vi "RPC Method package_service_method.vi"(8 "error in (no error)":errorcluster, 11 "ServiceName Template in":refnum<class "ServiceName Template.lvclass">) -> (0 "error out":errorcluster, 3 "ServiceName Template out":refnum<class "ServiceName Template.lvclass">)   [LabVIEW 2024, in "ServiceName Template.lvclass"]
uses:
  ServiceName Template.lvclass
  C:/serenial/oss/grpc-labview/labview source/gRPC lv Servicer/ServiceBase/ServiceBase.lvclass
  ServiceName Template.lvclass/ServiceName Template.ctl
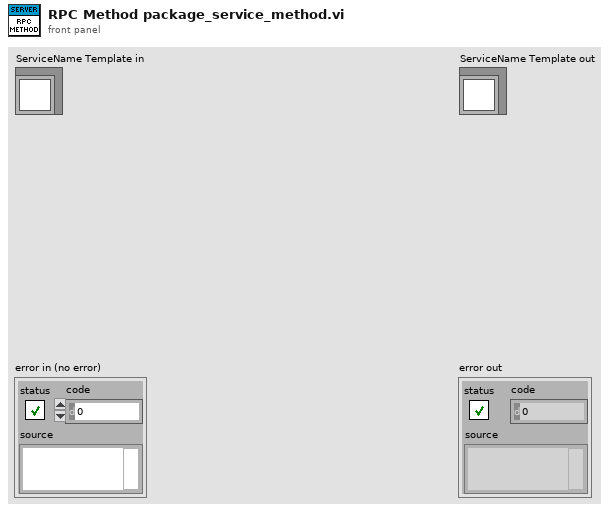
[diagram p1: front panel]
types:
  T1 = typedef "ServiceName Template.lvclass/Server Internal UEs.ctl" = cluster{"package_service_method Internal UE":refnum<user-event>}
  T2 = typedef "ServiceName Template.lvclass/Server gRPC UEs.ctl" = cluster{"package_service_method":refnum<user-event>}
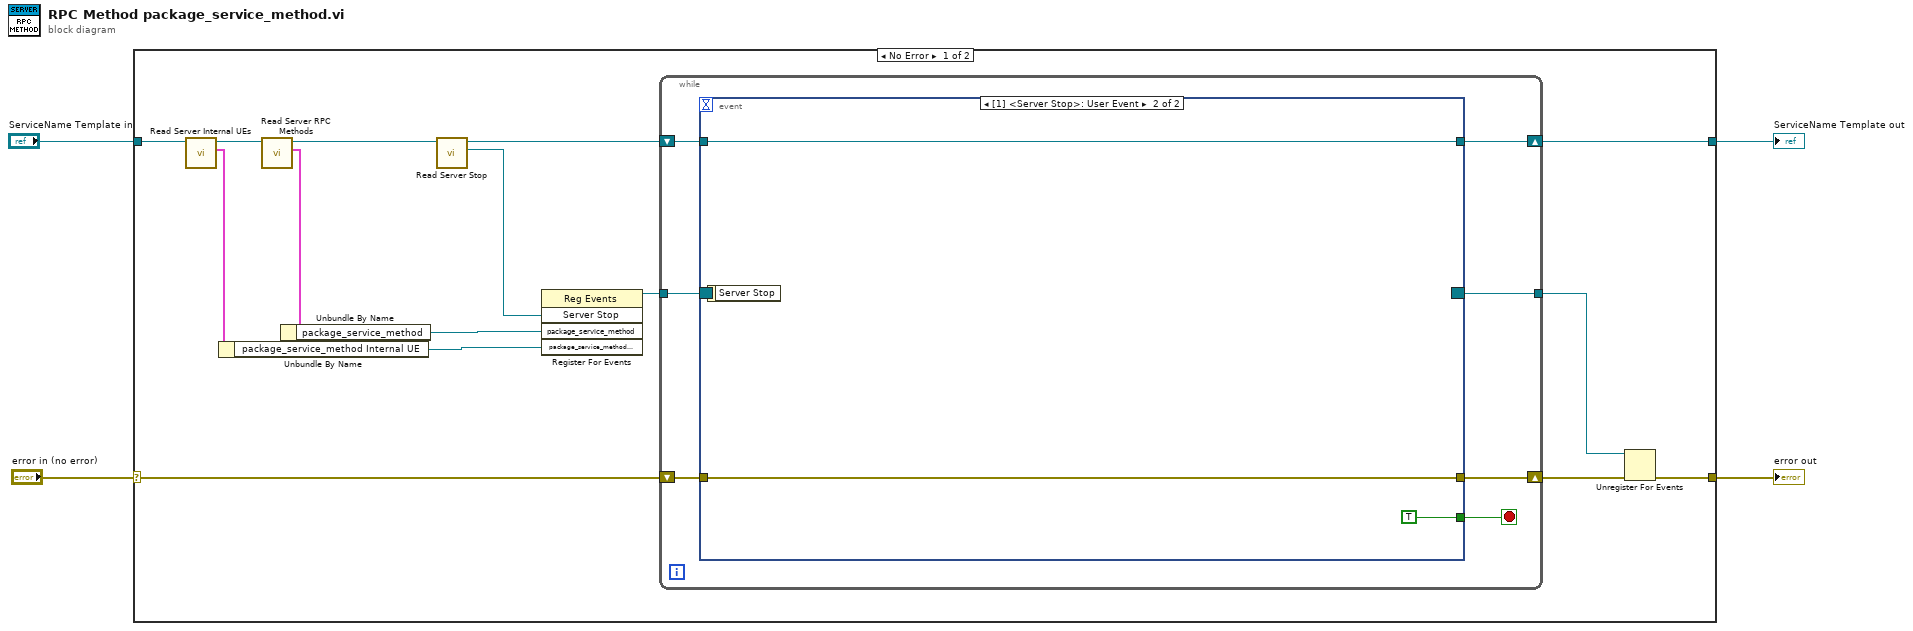
[diagram p0: block diagram]
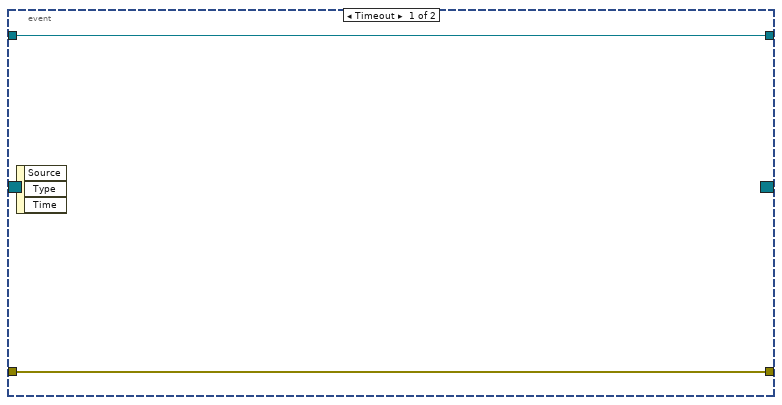
[diagram p2: hidden frame]
diagram:
  n1 = case shown="No Error" "error in (no error)" {
    selector: "error in (no error)" -> [w15 w33]
    tunnel: [w13 w33] -> w3
    tunnel: "ServiceName Template in" -> [w17 w32]
    tunnel: [w5 w32] -> w1
    frame No Error {
      n2 = call "Read Server Internal UEs.vi"("ServiceName Template in"=w17) -> ("Server Internal UEs"=w9:T1, "ServiceName Template out"=w16:refnum<class "ServiceName Template.lvclass">)  [unwired: 8 in, 1 out]
      n3 = Unbundle By Name ("Unbundle Internal UE")(w9) -> ("package_service_method Internal UE"=w8:refnum<user-event>)
      n4 = call "Read Server RPC Methods.vi"("ServiceName Template in"=w16) -> ("Server RPC Methods"=w11:T2, "ServiceName Template out"=w6:refnum<class "ServiceName Template.lvclass">)  [unwired: 8 in, 1 out]
      n5 = Unbundle By Name ("Unbundle gRPC UE")(w11) -> ("package_service_method"=w10:refnum<user-event>)
      n6 = call-dynamic "Read Server Stop.vi"("iService in"=w6) -> ("Server Stop"=w19:refnum<user-event>, "iService out"=w7:refnum<class "ServiceName Template.lvclass">)  [unwired: 8 in, 1 out]
      n7 = register-events(w19, w10, w8) -> (reference out=w18:refnum<event-registration>)  [unwired: 2 in, 1 out]
      n8 = while {
        tunnel: w18 -> [w26]
        tunnel: [w22] -> w12
        shift-right: [w23] -> w14
        shift-left: w15 -> [w24]
        shift-right: [w20] -> w5
        shift-left: w7 -> [w21]
        stop <- w25 stop-if-true
        n9 = event "RPC Method Event Structure" shown="[1] <Server Stop>: User Event" {
          selector: w26 -> [_ _]
          dyn-events: [_ _] -> w22
          timeout: _ -> [_ _]
          tunnel: [_ TRUE] -> w25
          tunnel: w24 -> [w28 w30]
          tunnel: [w28 w30] -> w23
          tunnel: w21 -> [w27 w29]
          tunnel: [w27 w29] -> w20
          event Timeout {
            n10 = event-data() -> ()  [unwired: 1 in, 3 out]
          }
          event User Event {
            n11 = event-data() -> ()  [unwired: 1 in, 1 out]
          }
        }
      }
      n12 = Unregister For Events(event registration refnum=w12, error in=w14) -> (error out=w13:errorcluster)
    }
    frame Error {
    }
  }
  "error out" <- w3
  "ServiceName Template out" <- w1
